vi "U16 logic test.vi"() -> ()   [LabVIEW 2013]
panel:
  in  "U16":u16 format="%b"
  out ".not. x?":u16 format="%b"
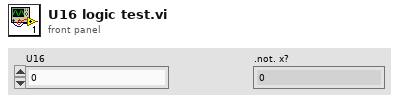
[diagram p1: front panel]
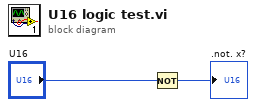
[diagram p0: block diagram]
diagram:
  n1 = Not(x="U16") -> (.not. x?=→".not. x?":u16)
